vi "Scale Label Linear.vi"(8 "error in (no error)":errorcluster, 9 "Scaling limits":cluster{"Y lower":dbl, "Y upper":dbl}, 10 "ymaxmin":cluster{"ymax":dbl, "ymin":dbl}, 11 "y":dbl) -> (0 "error out":errorcluster, 3 "y scaled":dbl)   [LabVIEW 2014]
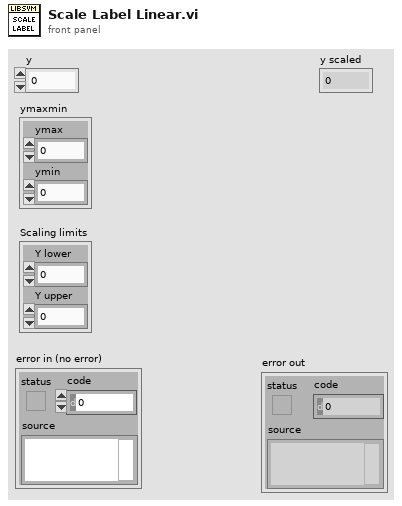
[diagram p1: front panel]
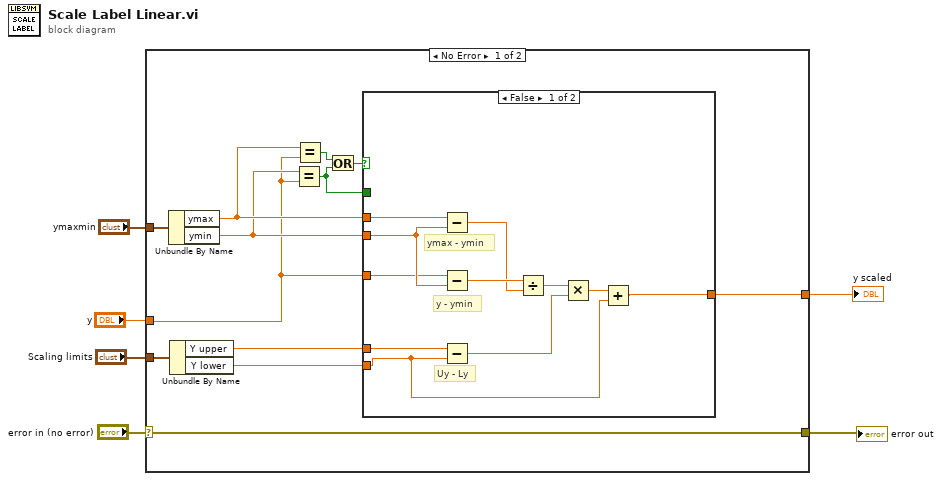
[diagram p0: block diagram]
diagram:
  n1 = case shown="No Error" "error in (no error)" {
    selector: "error in (no error)" -> [w11 w37]
    tunnel: [w11 w37] -> w6
    tunnel: "Scaling limits" -> [w17 _]
    tunnel: "y" -> [w8 _]
    tunnel: "ymaxmin" -> [w18 _]
    tunnel: [w7 nan] -> w1
    frame No Error {
      n2 = Unbundle By Name(w18) -> ("ymax"=w10:dbl, "ymin"=w9:dbl)
      n3 = Unbundle By Name(w17) -> ("Y upper"=w13:dbl, "Y lower"=w12:dbl)
      n4 = Equal?(x=w9, y=w8) -> (x = y?=w14:bool)
      n5 = Equal?(x=w10, y=w8) -> (x = y?=w16:bool)
      n6 = Or(x=w16, y=w14) -> (x .or. y?=w15:bool)
      n7 = case shown="False" w15 {
        tunnel: w14 -> [_ w33]
        tunnel: w13 -> [w21 w32]
        tunnel: w12 -> [w20 w31]
        tunnel: [w19 w30] -> w7
        tunnel: w10 -> [w24 _]
        tunnel: w9 -> [w23 _]
        tunnel: w8 -> [w22 _]
        frame False {
          # "ymax - ymin"
          # "y - ymin"
          # "Uy - Ly"
          n8 = Subtract(x=w24, y=w23) -> (x-y=w28:dbl)
          n9 = Subtract(x=w22, y=w23) -> (x-y=w29:dbl)
          n10 = Subtract(x=w21, y=w20) -> (x-y=w26:dbl)
          n11 = Divide(x=w29, y=w28) -> (x/y=w27:dbl)
          n12 = Multiply(x=w27, y=w26) -> (x*y=w25:dbl)
          n13 = Add(x=w25, y=w20) -> (x+y=w19:dbl)
        }
        frame True {
          n14 = case shown="True" w33 {
            tunnel: w32 -> [_ w35]
            tunnel: w31 -> [w34 _]
            tunnel: [w34 w35] -> w30
            frame False {
            }
            frame True {
            }
          }
        }
      }
    }
    frame Error {
    }
  }
  "error out" <- w6
  "y scaled" <- w1
